vi "Process Data.vi"(8 "error in":errorcluster, 11 "Client in":refnum<class "Client.lvclass">) -> (0 "error out":errorcluster, 3 "Client out":refnum<class "Client.lvclass">)   [LabVIEW 2014, in "Client.lvclass"]
uses:
  Client.lvclass
  Topic_class/Topic.lvclass
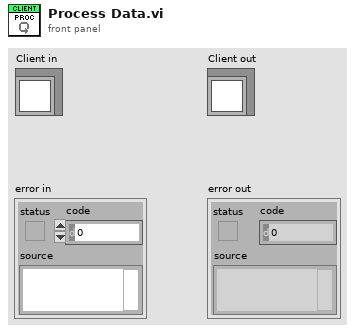
[diagram p1: front panel]
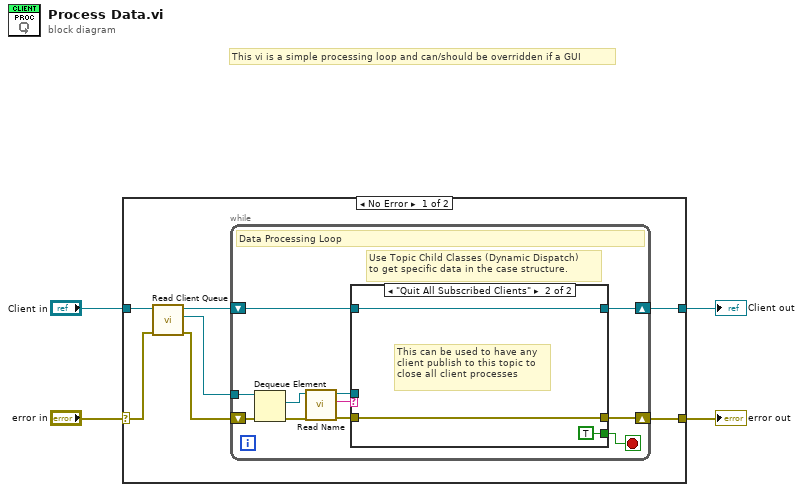
[diagram p0: block diagram]
diagram:
  # "This vi is a simple processing loop and can/should be overridden if a GUI"
  n1 = case shown="No Error" "error in" {
    selector: "error in" -> [w5 w29]
    tunnel: [w6 w29] -> w3
    tunnel: [w8 w28] -> w1
    tunnel: "Client in" -> [w11 w28]
    frame No Error {
      n2 = call-dynamic "Read Client Queue.vi"("error in"=w5, "Client in"=w11) -> ("error out"=w7:errorcluster, "Client Queue"=w10:refnum<queue>, "Client out"=w9:refnum<class "Client.lvclass">)  [unwired: 7 in]
      n3 = while {
        tunnel: w10 -> [w22]
        shift-right: [w14] -> w8
        shift-left: w9 -> [w15]
        shift-right: [w12] -> w6
        shift-left: w7 -> [w13]
        stop <- w16 stop-if-true
        # "Use Topic Child Classes (Dynamic Dispatch)\nto get specific data in the case structure."
        # "Data Processing Loop"
        n4 = Dequeue Element(queue=w22, error in (no error)=w13) -> (element=w20:refnum<class "Topic.lvclass">, error out=w21:errorcluster)  [unwired: 1 in, 2 out]
        n5 = call-dynamic "Read Name.vi"("error in"=w21, "Topic in"=w20) -> ("error out"=w18:errorcluster, "Name"=w19:string, "Topic out"=w17:refnum<class "Topic.lvclass">)  [unwired: 7 in]
        n6 = case shown="\"Quit All Subscribed Clients\"" w19 {
          tunnel: [_ TRUE] -> w16
          tunnel: w18 -> [w24 w26]
          tunnel: [w24 w26] -> w12
          tunnel: w17 -> [_ _]
          tunnel: w15 -> [w23 w25]
          tunnel: [w23 w25] -> w14
          frame Default {
          }
          frame "Quit All Subscribed Clients" {
            # "This can be used to have any\nclient publish to this topic to\nclose all client processes"
          }
        }
      }
    }
    frame Error {
    }
  }
  "error out" <- w3
  "Client out" <- w1
